vi "CAlex2_SetCuff_Thigh2.vi"(10 "Thigh Cuff Distance":dbl, 11 "Thigh Cuff Center from Knee":dbl) -> (2 "Thigh Cuff Low":T1={"BodyID"=0, "CoM(CuffCS)"={"Coord4"=[0.0, 0.0, 0.0, 1.0], "ID"=0}, "Mass(kg)"=0.0, "CablePts(CuffCS)"=[], "Cuff->Body"=[[1.0, 0.0, 0.0, 0.0], [0.0, 1.0, 0.0, 0.0], [0.0, 0.0, 1.0, 0.0], [0.0, 0.0, 0.0, 1.0]]}, 3 "Thigh Cuff High":T1={"BodyID"=0, "CoM(CuffCS)"={"Coord4"=[0.0, 0.0, 0.0, 1.0], "ID"=0}, "Mass(kg)"=0.0, "CablePts(CuffCS)"=[], "Cuff->Body"=[[1.0, 0.0, 0.0, 0.0], [0.0, 1.0, 0.0, 0.0], [0.0, 0.0, 1.0, 0.0], [0.0, 0.0, 0.0, 1.0]]})   [LabVIEW 2015, in "CAlex2.lvclass"]
uses:
  CAlex2.lvclass
  CableSerialChain/TypeDef/Cuff.ctl
  Body/PointOnBody.ctl
  <vilib>/Analysis/Matrix/Datatypes/RealMatrix.ctl
  <vilib>/Analysis/Matrix/NI_Matrix.lvlib
  Body/Bodies.lvclass
  CableSerialChain/CableSerialChain.lvclass
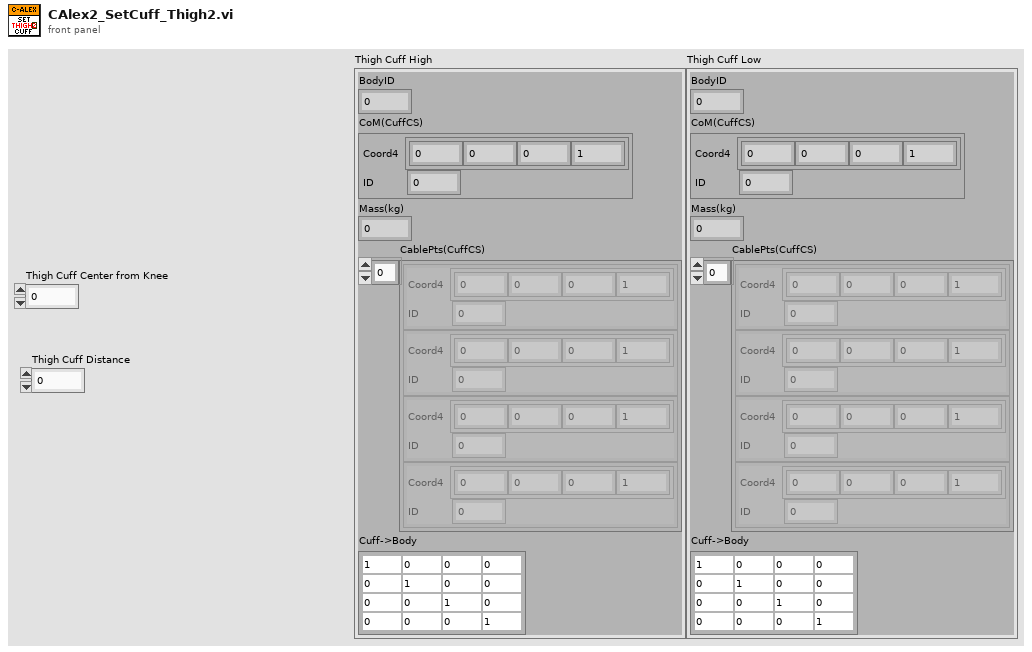
[diagram p1: front panel]
types:
  T1 = typedef "CableSerialChain.lvclass/Cuff.ctl" = cluster{"BodyID":i32, "CoM(CuffCS)":T2, "Mass(kg)":dbl, "CablePts(CuffCS)":T2[], "Cuff->Body":T3}
  T2 = typedef "Bodies.lvclass/PointOnBody.ctl" = cluster{"Coord4":dbl[], "ID":i32}
  T3 = typedef "NI_Matrix.lvlib/RealMatrix.ctl" = dbl[][]
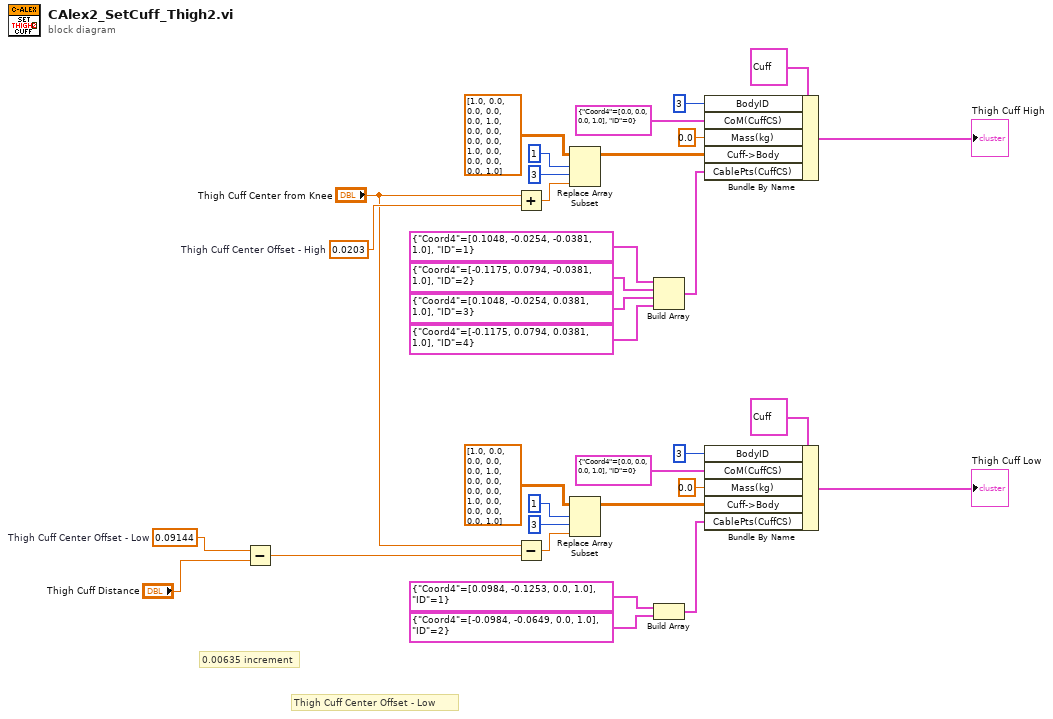
[diagram p0: block diagram]
diagram:
  w3 = 0.09144  # Thigh Cuff Center Offset - Low
  w19 = 0.0203  # Thigh Cuff Center Offset - High
  # "0.00635 increment"
  # "Thigh Cuff Center Offset - Low"
  n1 = Subtract(x=w3, y="Thigh Cuff Distance") -> (x-y=w2:dbl)
  n2 = Add(x="Thigh Cuff Center from Knee", y=w19) -> (x+y=w18:dbl)
  n3 = Subtract(x="Thigh Cuff Center from Knee", y=w2) -> (x-y=w17:dbl)
  n4 = Replace Array Subset(array=T3 [[1.0, 0.0, 0.0, 0.0], [0.0, 1.0, 0.0, 0.0], [0.0, 0.0, 1.0, 0.0], [0.0, 0.0, 0.0, 1.0]] ("Cuff->Leg"), new element=w18, index (row)=1, index (col)=3 ("index (row)")) -> (w28:T3)
  n5 = Replace Array Subset(array=T3 [[1.0, 0.0, 0.0, 0.0], [0.0, 1.0, 0.0, 0.0], [0.0, 0.0, 1.0, 0.0], [0.0, 0.0, 0.0, 1.0]] ("Cuff->Leg"), new element=w17, index (row)=1, index (col)=3 ("index (row)")) -> (w10:T3)
  n6 = Build Array(T2 {"Coord4"=[0.1048, -0.0254, -0.0381, 1.0], "ID"=1} ("CoM(CuffCS)"), T2 {"Coord4"=[-0.1175, 0.0794, -0.0381, 1.0], "ID"=2} ("CoM(CuffCS)"), T2 {"Coord4"=[0.1048, -0.0254, 0.0381, 1.0], "ID"=3} ("CoM(CuffCS)"), T2 {"Coord4"=[-0.1175, 0.0794, 0.0381, 1.0], "ID"=4} ("CoM(CuffCS)")) -> (w25:T2[])
  n7 = Build Array(T2 {"Coord4"=[0.0984, -0.1253, 0.0, 1.0], "ID"=1} ("CoM(CuffCS)"), T2 {"Coord4"=[-0.0984, -0.0649, 0.0, 1.0], "ID"=2} ("CoM(CuffCS)")) -> (w11:T2[])
  n8 = Bundle By Name(cluster=T1 {"BodyID"=0, "CoM(CuffCS)"={"Coord4"=[0.0, 0.0, 0.0, 1.0], "ID"=0}, "Mass(kg)"=0.0, "CablePts(CuffCS)"=[], "Cuff->Body"=[[1.0, 0.0, 0.0, 0.0], [0.0, 1.0, 0.0, 0.0], [0.0, 0.0, 1.0, 0.0], [0.0, 0.0, 0.0, 1.0]]} ("Cuff Design"), "BodyID"=3, "CoM(CuffCS)"=T2 {"Coord4"=[0.0, 0.0, 0.0, 1.0], "ID"=0}, "Mass(kg)"=0.0, "Cuff->Body"=w28, "CablePts(CuffCS)"=w25) -> (→"Thigh Cuff High":T1)
  n9 = Bundle By Name(cluster=T1 {"BodyID"=0, "CoM(CuffCS)"={"Coord4"=[0.0, 0.0, 0.0, 1.0], "ID"=0}, "Mass(kg)"=0.0, "CablePts(CuffCS)"=[], "Cuff->Body"=[[1.0, 0.0, 0.0, 0.0], [0.0, 1.0, 0.0, 0.0], [0.0, 0.0, 1.0, 0.0], [0.0, 0.0, 0.0, 1.0]]} ("Cuff Design"), "BodyID"=3, "CoM(CuffCS)"=T2 {"Coord4"=[0.0, 0.0, 0.0, 1.0], "ID"=0}, "Mass(kg)"=0.0, "Cuff->Body"=w10, "CablePts(CuffCS)"=w11) -> (→"Thigh Cuff Low":T1)
